vi "Create Paragraph for Cell.vi"(0 "Image to Add [ ]":T7, 2 "PDF Report IN":refnum<class "PDF Report Class.lvclass">, 5 "String":string, 7 "Column Width (points)":dbl, 11 "error in (no error)":errorcluster, 13 "Row format with ref":T6, 14 "i":i32) -> (4 "Valid Image?":bool, 6 "Modify Padding?":bool, 8 "Font Size":sgl, 10 "Paragraph refnum":refnum<k24>, 15 "error out":errorcluster)   [LabVIEW 2019, in "Exaprom PDF.lvlib"]
doc: "Version 2.0\nDeveloped by Jean-Marc Simard\nCopyright © 2010, Exaprom Inc.\nAll rights reserved.\nLicense: BSD\n\nWith iTextSharp 4.1.6 (http://itextsharp.sourceforge.net)\nunder Mozilla Public License Version 1.1\n(http://www.mozilla.org/MPL/MPL-1.1.html)"
uses:
  Controls/General Controls/Image to Add refnum [ ].ctl
  C:/work/niobrara_lv/labview pdf writer fixing/DLL/itextsharp.dll
  DLL/itextsharp.dll
  Controls/Table Controls/Cell Cluster.ctl
  Controls/Text Controls/Unicode/Type and run direction.ctl
  Controls/Table Controls/Cell Alignment 20px.ctl
  Controls/Table Controls/Text vertical arrangement.ctl
  Controls/Font Controls/Font size.ctl
  LV Class/PDF Report Class/PDF Report Class.lvclass
  Controls/Text Controls/Phrase or paragraph.ctl
  Controls/Image Controls/Image Scale Type.ctl
  Exaprom PDF.lvlib
  LV Class/Fonts Class/Font Class.lvclass
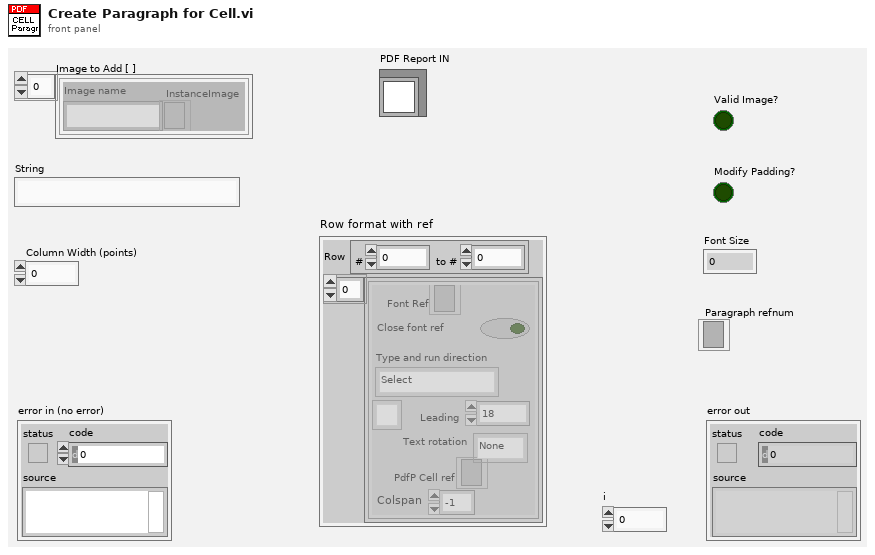
[diagram p1: front panel]
types:
  T1 = typedef "Exaprom PDF.lvlib/Cell Cluster.ctl" = cluster{"Font Ref":refnum<k24>, "Close font ref":bool, "Type and run direction":T2, "Cell Alignment":T3, "Text rotation":T4, "Leading":T5, "PdfP Cell ref":refnum<k24>, "Colspan":i8}
  T2 = typedef "Exaprom PDF.lvlib/Type and run direction.ctl" = enum16{"Select", "ASCII", "UTF-16", "UTF-16 (default)", "UTF-16 (LTR)", "UTF-16 (RTL)"}
  T3 = typedef "Exaprom PDF.lvlib/Cell Alignment 20px.ctl" = u16
  T4 = typedef "Exaprom PDF.lvlib/Text vertical arrangement.ctl" = enum16{"None", "Clockwise", "Counterclockwise"}
  T5 = typedef "Exaprom PDF.lvlib/Font size.ctl" = sgl
  T6 = cluster{"Row":cluster{"#":i16, "to #":i16}, "Cell [ ]":T1[]}
  T7 = typedef "Exaprom PDF.lvlib/Image to Add refnum [ ].ctl" = cluster{"Image name":string, "InstanceImage":refnum<k24>}[]
  T8 = typedef "Exaprom PDF.lvlib/Phrase or paragraph.ctl" = enum16{"Add to Phrase", "Add to Paragraph", "Create Phrase", "Create Paragraph"}
  T9 = typedef "Exaprom PDF.lvlib/Image Scale Type.ctl" = enum16{"%", "Height", "Width"}
  T10 = typedef "Exaprom PDF.lvlib/Texte alignement.ctl" = enum16{"Select", "CENTER", "JUSTIFY", "LEFT", "RIGHT"}
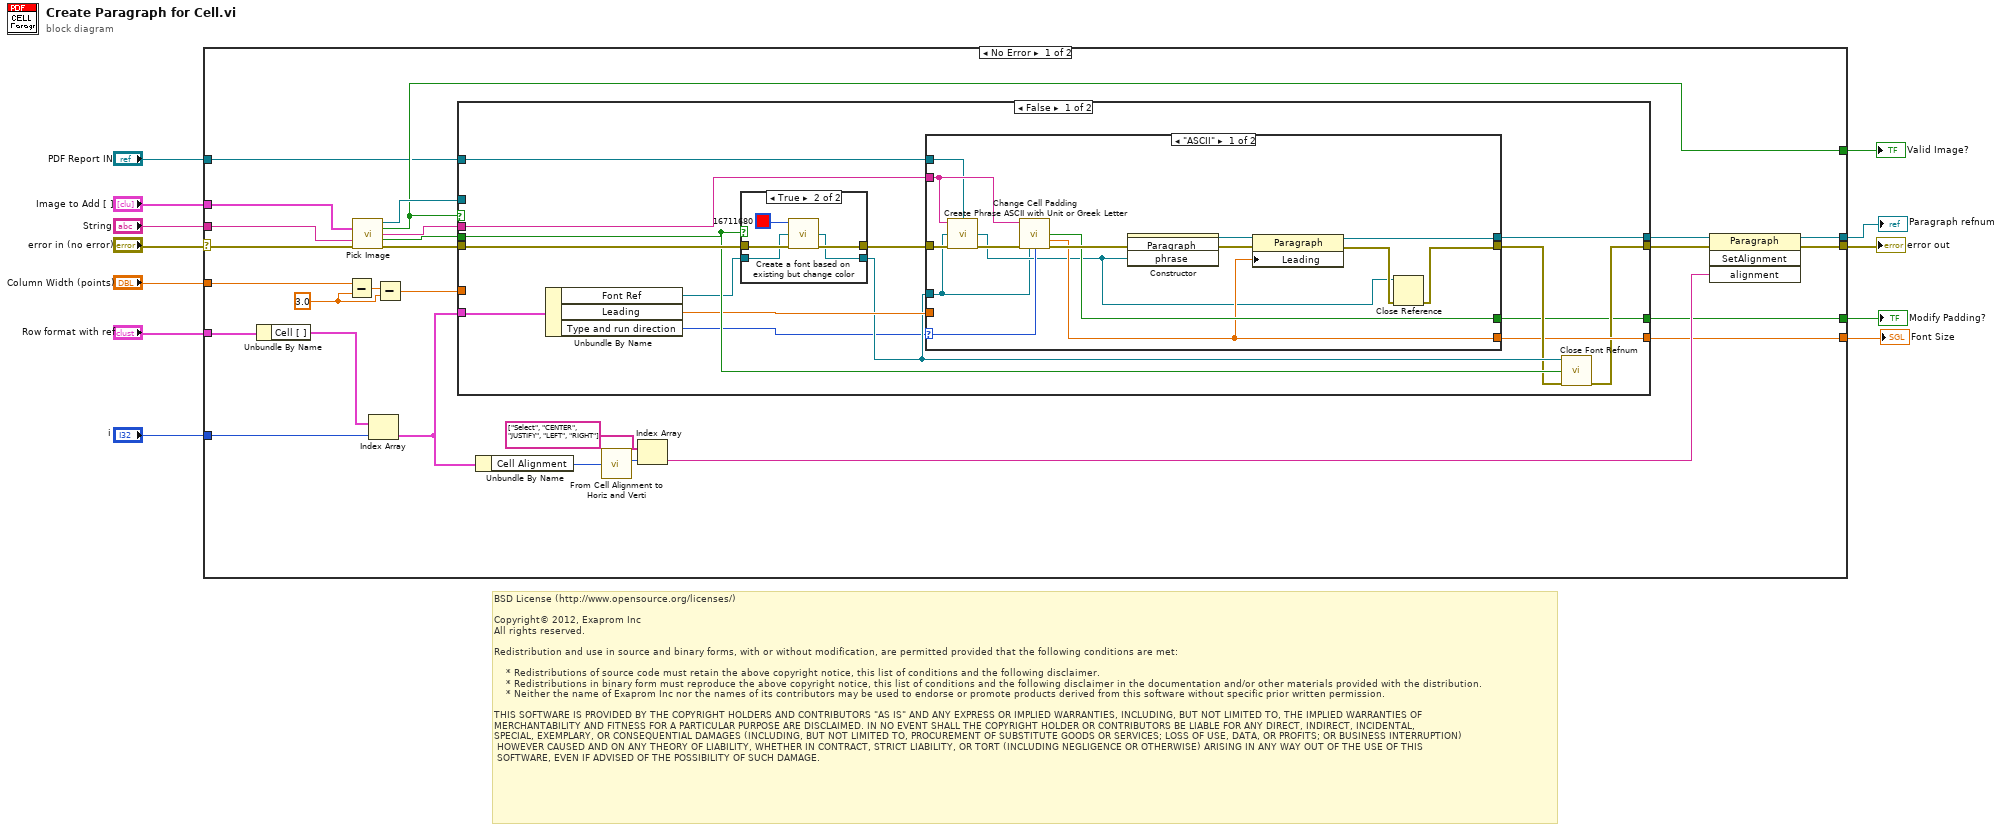
[diagram p0: block diagram]
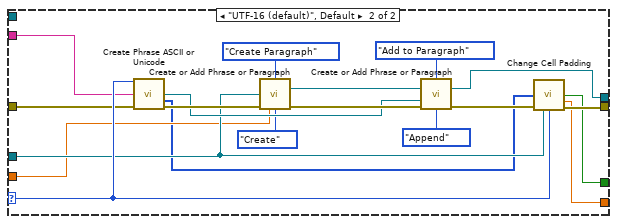
[diagram p2: hidden frame]
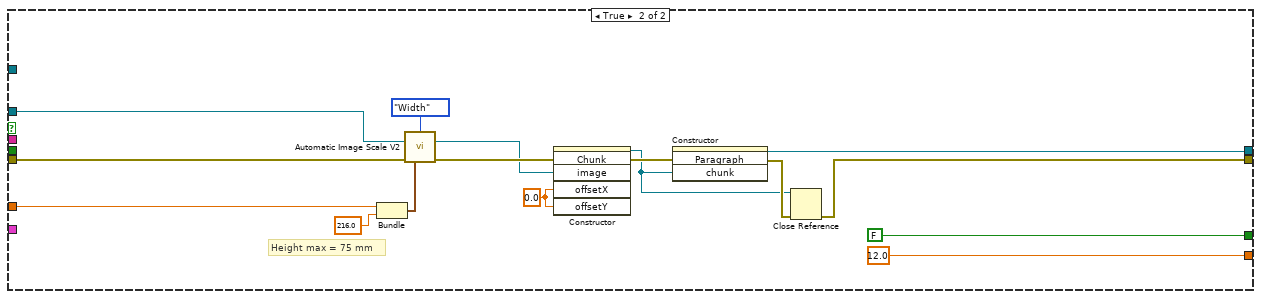
[diagram p4: hidden frame]
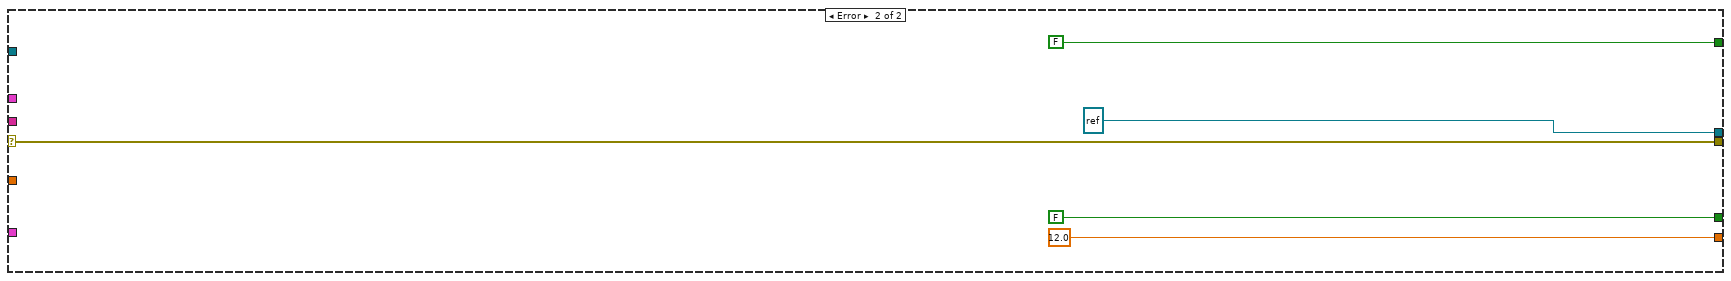
[diagram p5: hidden frame]
diagram:
  # "BSD License (http://www.opensource.org/licenses/)\n\nCopyright© 2012, Exaprom Inc\nAll rights reserved.\n\nRedistribution and use in source and binary forms, with or without modification, are permitted provided that the following conditions are met:\n\n    * Redistributions of source code must retain the above copyright notice, this list of conditions and the following disclaimer.\n    * Redistributions in binary form must reproduce the above copyright notice, this list of conditions and the following disclaimer in the documentation and/or other materials provided with the distribution.\n    * Neither the name of Exaprom Inc nor the names of its contributors may be used to endorse or promote products derived from this software without specific prior written permission.\n\nTHIS SOFTWARE IS PROVIDED BY THE COPYRIGHT HOLDERS AND CONTRIBUTORS \"AS IS\" AND ANY EXPRESS OR IMPLIED WARRANTIES, INCLUDING, BUT NOT LIMITED TO, THE IMPLIED WARRANTIES OF \nMERCHANTABILITY AND FITNESS FOR A PARTICULAR PURPOSE ARE DISCLAIMED. IN NO EVENT SHALL THE COPYRIGHT HOLDER OR CONTRIBUTORS BE LIABLE FOR ANY DIRECT, INDIRECT, INCIDENTAL,\nSPECIAL, EXEMPLARY, OR CONSEQUENTIAL DAMAGES (INCLUDING, BUT NOT LIMITED TO, PROCUREMENT OF SUBSTITUTE GOODS OR SERVICES; LOSS OF USE, DATA, OR PROFITS; OR BUSINESS INTERRUPTION)\n HOWEVER CAUSED AND ON ANY THEORY OF LIABILITY, WHETHER IN CONTRACT, STRICT LIABILITY, OR TORT (INCLUDING NEGLIGENCE OR OTHERWISE) ARISING IN ANY WAY OUT OF THE USE OF THIS\n SOFTWARE, EVEN IF ADVISED OF THE POSSIBILITY OF SUCH DAMAGE."
  n1 = case shown="No Error" "error in (no error)" {
    selector: "error in (no error)" -> [w29 w116]
    tunnel: [w21 w116] -> w11
    tunnel: "String" -> [w30 _]
    tunnel: "Image to Add [ ]" -> [w31 _]
    tunnel: "Column Width (points)" -> [w39 _]
    tunnel: "i" -> [w23 _]
    tunnel: "Row format with ref" -> [w16 _]
    tunnel: [w20 FALSE] -> w6
    tunnel: [w19 sgl 12.0 ("Size")] -> w5
    tunnel: [w18 FALSE ("Valid Image?")] -> w4
    tunnel: [w17 refnum<k24> refnum ("new reference")] -> w3
    tunnel: "PDF Report IN" -> [w13 _]
    frame No Error {
      w37 = sgl 3.0 ("t")
      n2 = Unbundle By Name(w16) -> ("Cell [ ]"=w24:T1[])
      n3 = Subtract(x=w39, y=w37) -> (x-y=w38:dbl)
      n4 = call "Pick Image.vi"("Image to Add [ ]"=w31, "String"=w30, "error in (no error)"=w29) -> ("InstanceImage"=w27:refnum<k24>, "Valid Image?"=w18:bool, "String OUT"=w26:string, "Change Font Color?"=w25:bool, "error out"=w28:errorcluster)  [unwired: 8 out]
      n5 = Index Array(array=w24, index=w23) -> (element=w22:T1)
      n6 = Subtract(x=w38, y=w37) -> (x-y=w36:dbl)
      n7 = case shown="False" w18 {
        tunnel: w28 -> [w52 w97]
        tunnel: w27 -> [_ w96]
        tunnel: w36 -> [_ w111]
        tunnel: w25 -> [w51 _]
        tunnel: [w43 w103] -> w34
        tunnel: [w53 w107] -> w33
        tunnel: w26 -> [w47 _]
        tunnel: [w42 FALSE] -> w20
        tunnel: [w44 sgl 12.0 ("Size")] -> w19
        tunnel: w22 -> [w50 _]
        tunnel: w13 -> [w40 _]
        frame False {
          n8 = Unbundle By Name(w50) -> ("Font Ref"=w49:refnum<k24>, "Leading"=w48:T5, "Type and run direction"=w41:T2)
          n9 = case shown="True" w51 {
            tunnel: w52 -> [w89 w95]
            tunnel: w49 -> [w90 w94]
            tunnel: [w89 w93] -> w54
            tunnel: [w90 w92] -> w46
            frame False {
            }
            frame True {
              n10 = call "Create a font based on existing but change color.vi"("Color"=u32 16711680, "Font refnum"=w94, "error in (no error)"=w95) -> ("Font new color refnum"=w92:refnum<k24>, "error out"=w93:errorcluster)  [unwired: 11 in]
            }
          }
          n11 = case shown="\"ASCII\"" w41 {
            selector: w41 -> [w68 w75]
            tunnel: w54 -> [w60 w72]
            tunnel: [w64 w76] -> w53
            tunnel: w48 -> [_ w73]
            tunnel: w47 -> [w57 w71]
            tunnel: [w62 w79] -> w45
            tunnel: w46 -> [w56 w74]
            tunnel: [w67 w77] -> w42
            tunnel: [w61 w78] -> w44
            tunnel: w40 -> [w55 _]
            frame "ASCII" {
              n12 = call "Create Phrase ASCII with Unit or Greek Letter.vi"("Text"=w57, "PDF Report IN"=w55, "Cell Font Ref"=w56, "error in (no error)"=w60) -> ("Phrase refnum"=w58:refnum<k24>, "error out"=w59:errorcluster)  [unwired: 10 in]
              n13 = call "Change Cell Padding.vi"("String"=w57, "error in (no error)"=w59, "Font"=w56, "Type and run direction"=w68) -> ("Change cell padding?"=w67:bool, "Size"=w61:sgl, "error out duplicate"=w69:errorcluster)  [unwired: 9 in]
              n14 = constructor class="Paragraph"(error in=w69, "phrase"=w58) -> (reference out=w66:refnum<k24>, error out=w65:errorcluster)  [unwired: 2 in, 2 out]
              n15 = property class="Paragraph"(reference=w66, error in=w65, "Leading"=w61) -> (reference out=w64:refnum<k24>, error out=w63:errorcluster)
              n16 = Close Reference(reference=w58, error in (no error)=w63) -> (error out=w62:errorcluster)
            }
            frame "UTF-16 (default)", Default {
              n17 = call "Create Phrase ASCII or Unicode.vi"("Character type"=w75, "Text"=w71, "error in (no error)"=w72) -> ("Phrase refnum"=w83:refnum<k24>, "Char U16 [ ]"=w70:u16[], "error out"=w88:errorcluster)  [unwired: 10 in]
              n18 = call "Create or Add Phrase or Paragraph.vi"("Phrase or paragraph"=Phrase_or_paragraph."Create Paragraph", "Font refnum"=w74, "error in (no error)"=w88, "Leading"=w73, "Only"=enum16{"Create", "Append"}."Create") -> ("Paragraph refnum OUT"=w84:refnum<k24>, "error out"=w87:errorcluster)  [unwired: 8 in, 1 out]
              n19 = call "Create or Add Phrase or Paragraph.vi"("Phrase or paragraph"=Phrase_or_paragraph."Add to Paragraph", "Paragraph refnum IN"=w84, "value"=w83, "error in (no error)"=w87, "Only"=enum16{"Create", "Append"}."Append") -> ("Paragraph refnum OUT"=w76:refnum<k24>, "error out"=w80:errorcluster)  [unwired: 8 in, 1 out]
              n20 = call "Change Cell Padding.vi"("String (Char U16 [ ])"=w70, "error in (no error)"=w80, "Font"=w74, "Type and run direction"=w75) -> ("Change cell padding?"=w77:bool, "Size"=w78:sgl, "error out duplicate"=w79:errorcluster)  [unwired: 9 in]
            }
          }
          n21 = call "Close Font Refnum.vi"("Font Refnum"=w46, "Close ?"=w51, "error in (no error)"=w45) -> ("error out"=w43:errorcluster)  [unwired: 12 in]
        }
        frame True {
          w108 = sgl 0.0 ("offsetX")
          # "Height max = 75 mm"
          n22 = Bundle(w111, sgl 216.0) -> (w109:cluster{dbl, sgl})  [unwired: 1 out]
          n23 = call "Automatic Image Scale V2.vi"("Scale Type"=Image_Scale_Type."Width", "GetInstanceImage IN"=w96, "error in (no error)"=w97, "Box"=w109) -> ("GetInstanceImage OUT"=w98:refnum<k24>, "error out"=w99:errorcluster)  [unwired: 7 in, 3 out]
          n24 = constructor class="Chunk"(error in=w99, "image"=w98, "offsetX"=w108, "offsetY"=w108) -> (reference out=w104:refnum<k24>, error out=w106:errorcluster)  [unwired: 2 in, 4 out]
          n25 = constructor class="Paragraph"(error in=w106, "chunk"=w104) -> (reference out=w107:refnum<k24>, error out=w105:errorcluster)  [unwired: 2 in, 2 out]
          n26 = Close Reference(reference=w104, error in (no error)=w105) -> (error out=w103:errorcluster)
        }
      }
      n27 = Unbundle By Name(w22) -> ("Cell Alignment"=w32:T3)
      n28 = call "From Cell Alignment to Horiz and Verti.vi"("Cell Alignment"=w32) -> ("Horizontal Alignment"=w15:T10)  [unwired: 6 in, 1 out]
      n29 = Index Array(array=string[] ["Select", "CENTER", "JUSTIFY", "LEFT", "RIGHT"] ("Strings []"), index=w15) -> (element=w35:string)
      n30 = invoke class="Paragraph" method="SetAlignment"(reference=w33, error in=w34, "alignment"=w35) -> (reference out=w17:refnum<k24>, error out=w21:errorcluster)  [unwired: 1 in, 2 out]
    }
    frame Error {
    }
  }
  "error out" <- w11
  "Modify Padding?" <- w6
  "Font Size" <- w5
  "Valid Image?" <- w4
  "Paragraph refnum" <- w3
